vi "Iterate Animation.vi"(9 "Animation":T1, 10 "Color":u32(colorbox)=6618880, 11 "Index":i32) -> (3 "Raw Data":u8[](array[numeric]))   [LabVIEW 2019, in "LED Matrix Host.lvlib"]
uses:
  LED Matrix Host.lvlib
  Controls/Animation.ctl
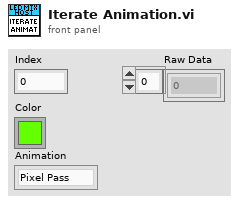
[diagram p1: front panel]
types:
  T1 = typedef "LED Matrix Host.lvlib/Animation.ctl" = enum16{"Pixel Pass", "Columns Pass", "Rows Pass", "Frame Pass"}
  T2 = typedef "LED Matrix Host.lvlib/Frame.ctl" = cluster{"Matrix":u32[][]}
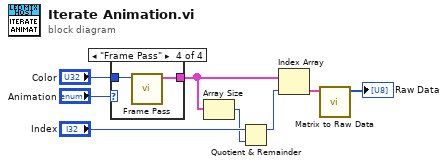
[diagram p0: block diagram]
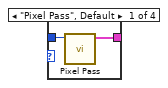
[diagram p2: hidden frame]
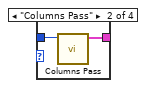
[diagram p3: hidden frame]
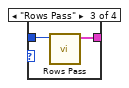
[diagram p4: hidden frame]
diagram:
  n1 = case shown="\"Frame Pass\"" "Animation" {
    tunnel: [w10 w11 w13 w15] -> w2
    tunnel: "Color" -> [w9 w12 w14 w16]
    frame "Pixel Pass", Default {
      n2 = call "Pixel Pass.vi"("Color Box"=w9) -> ("Frames"=w10:T2[])  [unwired: 10 in]
    }
    frame "Columns Pass" {
      n3 = call "Columns Pass.vi"("Color Box"=w12) -> ("Frames"=w11:T2[])  [unwired: 10 in]
    }
    frame "Rows Pass" {
      n4 = call "Rows Pass.vi"("Color Box"=w14) -> ("Frames"=w13:T2[])  [unwired: 10 in]
    }
    frame "Frame Pass" {
      n5 = call "Frame Pass.vi"("Color Box"=w16) -> ("Frames"=w15:T2[])  [unwired: 10 in]
    }
  }
  n6 = Array Size(array=w2) -> (size(s)=w1:i32)
  n7 = Quotient & Remainder(x="Index", y=w1) -> (x-y*floor(x/y)=w3:i32)  [unwired: 1 out]
  n8 = Index Array(array=w2, index=w3) -> (element=w7:T2)
  n9 = call "Matrix to Raw Data.vi"("Matrix"=w7) -> ("Raw Data"=→"Raw Data":u8[])  [unwired: 10 in]
